vi "InitSetup.vi"() -> ()   [LabVIEW 2023]
uses:
  <vilib>/Utility/error.llb/Error Cluster From Error Code.vi
  <vilib>/ErrorRing/Error Ring.xnode
panel:
  out "M9347 Status":string="Not Initilized"
  out "Chassis Status OK":bool
  out "error out":errorcluster {"code" format="%.0x"}
  in  "resource name":string="PXI0::25-0.0::INSTR" caption="PXI Chassis resource string"
  in  "M9300A resource string":string="PXI0::22-0.0::INSTR"
  in  "Port setting":T1={"Ch1"=TRUE, "Ch2"=FALSE, "Ch3"=FALSE, "Ch4"=FALSE, "Ch5"=FALSE, "backplane out"=TRUE, "10MHz out"=FALSE, "OCXO out"=FALSE, "bp Ref"=TRUE, "External Ref"=FALSE}
  # "This VI check the setup status and setup necessary things\nCheck the PXI chassis use timing module, and no alarm on the clock\nInitialize M9300 timing module\nInitialize M9347 LO"
  # "This program can be closed \nafter the M9347 is initialized."
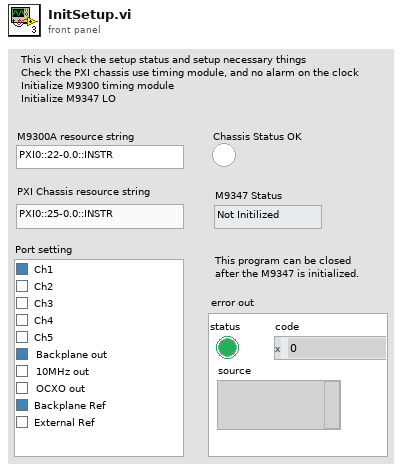
[diagram p1: front panel]
types:
  T1 = cluster{"Ch1":bool, "Ch2":bool, "Ch3":bool, "Ch4":bool, "Ch5":bool, "backplane out":bool, "10MHz out":bool, "OCXO out":bool, "bp Ref":bool, "External Ref":bool}
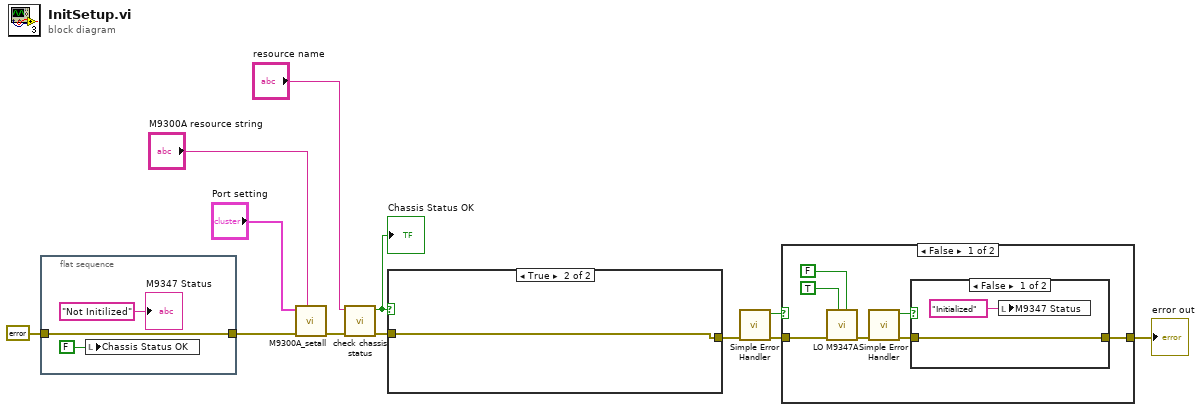
[diagram p0: block diagram]
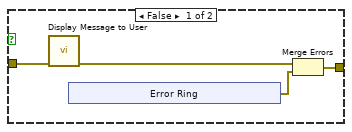
[diagram p4: hidden frame]
diagram:
  n1 = flat-sequence {
    tunnel: [w15] -> w3
    tunnel: errorcluster {"status"=FALSE, "code"=0, "source"=""} ("error in (no error)") -> [w15]
    frame #0 {
      n2 = local write "Chassis Status OK"(FALSE ("Chassis Status OK")) -> ()
      "M9347 Status" <- "Not Initilized" ("M9347 Status")
    }
  }
  n3 = call "M9300A_setall.vi"("resource string"="M9300A resource string", "error in (no error)"=w3, "Port setting"="Port setting") -> ("error out"=w9:errorcluster)  [unwired: 8 in]
  n4 = call "check chassis status.vi"("error in (no error)"=w9, "resource name"="resource name") -> ("error out"=w7:errorcluster, "Status OK"=w8:bool)  [unwired: 8 in]
  "Chassis Status OK" <- w8
  n5 = case shown="True" w8 {
    tunnel: w7 -> [w19 w25]
    tunnel: [w16 w25] -> w6
    frame False {
      n6 = call "Display Message to User"("error in (no error)"=w19) -> ("error out"=w18:errorcluster)  [unwired: 9 in, 1 out]
      n7 = xnode "Error Ring"() -> ("error out"=w17:errorcluster)
      n8 = Merge Errors(w18, w17) -> (w16:errorcluster)
    }
    frame True {
    }
  }
  n9 = call <vilib>:"Simple Error Handler.vi"("error in (no error)"=w6) -> ("error?"=w5:bool, "error out"=w4:errorcluster)  [unwired: 4 in, 3 out]
  n10 = case shown="False" w5 {
    tunnel: [w26 w36] -> w1
    tunnel: w4 -> [w30 w36]
    frame False {
      n11 = call "LO M9347A.vi"("Exec"=FALSE, "Init"=TRUE, "error in (no error)"=w30) -> ("error out"=w27:errorcluster)  [unwired: 8 in]
      n12 = call <vilib>:"Simple Error Handler.vi"("error in (no error)"=w27) -> ("error?"=w28:bool, "error out"=w29:errorcluster)  [unwired: 4 in, 3 out]
      n13 = case shown="False" w28 {
        tunnel: w29 -> [w34 w35]
        tunnel: [w34 w35] -> w26
        frame False {
          n14 = local write "M9347 Status"("Initialized") -> ()
        }
        frame True {
        }
      }
    }
    frame True {
    }
  }
  "error out" <- w1
